vi "NI VeriStand - Get Custom Device Version.vi"(8 "error in (no error)":errorcluster, 11 "Device Ref in":T1 format="%.0x") -> (0 "error out":errorcluster, 2 "Value":string, 3 "Device Ref out":T1 format="%.0x")   [LabVIEW 2020, in "Custom Device API.lvlib"]
doc: "Returns version information for a custom device. You can use the <B>Value</B> string this VI returns as an input to code that specifies different actions based on the version. For example, you can check the version string to determine whether to update device dependencies or, if you are bringing a custom device forward into a new version of NI VeriStand, to determine whether to run mutation code."
uses:
  <vilib>/NI VeriStand/Custom Device API/Custom Device API.lvlib
  <vilib>/NI VeriStand/Custom Device API/Custom Device Item Ref.ctl
  ff6269ed-d371-4d62-9528-9cf680979576.vi
  <vilib>/NI VeriStand/Custom Device API/Custom Device Offline Path.vi
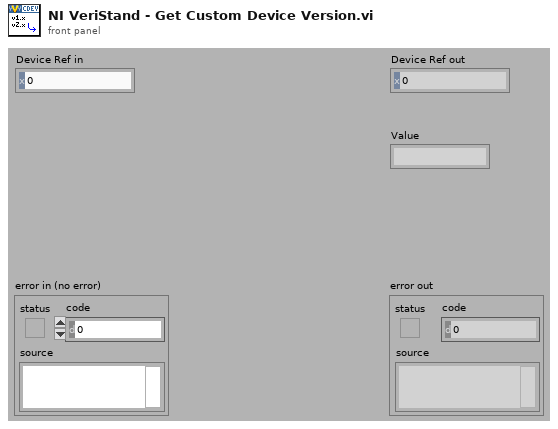
[diagram p1: front panel]
types:
  T1 = typedef "Custom Device API.lvlib/Custom Device Item Ref.ctl" = u64
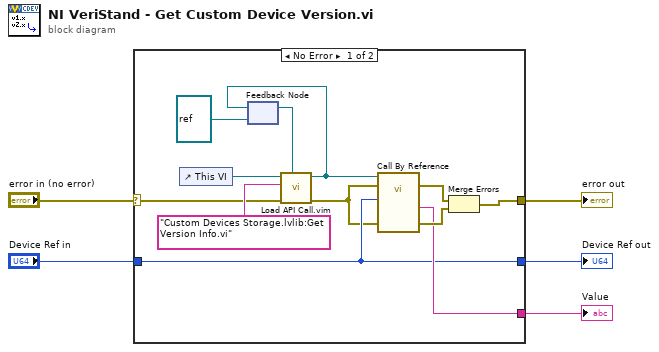
[diagram p0: block diagram]
diagram:
  n1 = case shown="No Error" "error in (no error)" {
    selector: "error in (no error)" -> [w7 w19]
    tunnel: "Device Ref in" -> [w14 w18]
    tunnel: [w16 w19] -> w4
    tunnel: [w14 w18] -> w3
    tunnel: [w15 _] -> w2
    frame No Error {
      n2 = control-ref of="This VI"() -> (w12:refnum<vi>)
      n3 = feedback #1(refnum<vi> refnum ("type specifier VI Refnum (for type only)")) -> (w13:refnum<vi>)
      n4 = call "Load API Call.vim"("VI reference in"=w13, "error in (no error)"=w7, "VI qualified name"="Custom Devices Storage.lvlib:Get Version Info.vi", "Caller VI ref"=w12) -> ("error out"=w8:errorcluster, "VI reference"=w11:refnum<vi>)  [unwired: 6 in]
      n5 = feedback-in #1(w11) -> ()
      n6 = call-by-ref "?"(reference=w11, error in=w8, 8:"error in (no error)"=w8, "Device Ref in"=w14) -> (error out=w6:errorcluster, 0:"error out"=w17:errorcluster, "Value"=w15:string)  [unwired: 7 in, 2 out]
      n7 = Merge Errors(w6, w17) -> (w16:errorcluster)
    }
    frame Error {
    }
  }
  "Device Ref out" <- w3
  "error out" <- w4
  "Value" <- w2
